vi "FollowAttacker.vi"(8 "error in (no error)":errorcluster, 9 "Game":refnum<class "Game.lvclass">, 10 "Robot":refnum<class "Robot.lvclass">, 11 "FollowAttackerSkill in":refnum<class "FollowAttackerSkill.lvclass">) -> (0 "error out":errorcluster, 2 "Robot out":refnum<class "Robot.lvclass">, 3 "FollowAttackerSkill out":refnum<class "FollowAttackerSkill.lvclass">)   [LabVIEW 2018, in "FollowAttackerSkill.lvclass"]
uses:
  FollowAttackerSkill.lvclass
  Robot_class/Robot.lvclass
  C:/Users/nicolas.oliveira/roboime/SSL_AI/Object_class/Object.lvclass
  Game_class/Game.lvclass
  Utilities_class/Utilities.lvclass
  Game_class/Game.lvclass/Game.ctl
  Team_class/Team.lvclass/Team.ctl
  Parameters_class/Parameters.lvclass/Parameters.ctl
  Events_class/Events.lvclass/Events.ctl
  Object_class/Object.lvclass/Object.ctl
  Robot_class/Robot.lvclass/Robot.ctl
  Robot_class/roles.ctl
  Object_class/Read x.vi
  Object_class/Read y.vi
  Robot_class/Read role.vi
  Robot_class/Read orientation.vi
  Game_class/Read EventsRef.vi
  Game_class/Read BallRef.vi
  Game_class/Read FieldRef.vi
  Game_class/Read OffensiveTeam.vi
  Game_class/Read Parameters.lvclass.vi
  Parameters_class/Read AttakingOurselves.vi
  Parameters_class/Read DistanceInFrontOfAttacker.vi
  Parameters_class/Read DistanceBehindAttacker.vi
  Team_class/Read RobotRef.vi
  Events_class/Read ball_inside_enemy_goalie_area.vi
  Events_class/Read ball_inside_our_goalie_area.vi
  Robot_class/Write dest_x.vi
  Robot_class/Write dest_y.vi
  Robot_class/Write dest_orientation.vi
  Robot_class/Write dest_vel.vi
  Ally_class/Ally.lvclass
  C:/Users/nicolas.oliveira/roboime/SSL_AI/Team_class/Team.lvclass
  Ball_class/Ball.lvclass
  Events_class/Events.lvclass
  Field_class/Field.lvclass
  Parameters_class/Parameters.lvclass
panel:
  out "sentido":dbl
  out "Yattacker":dbl
  out "Xattacker":dbl
  in  "Upper limit":dbl=300.0 format="%#_13g"
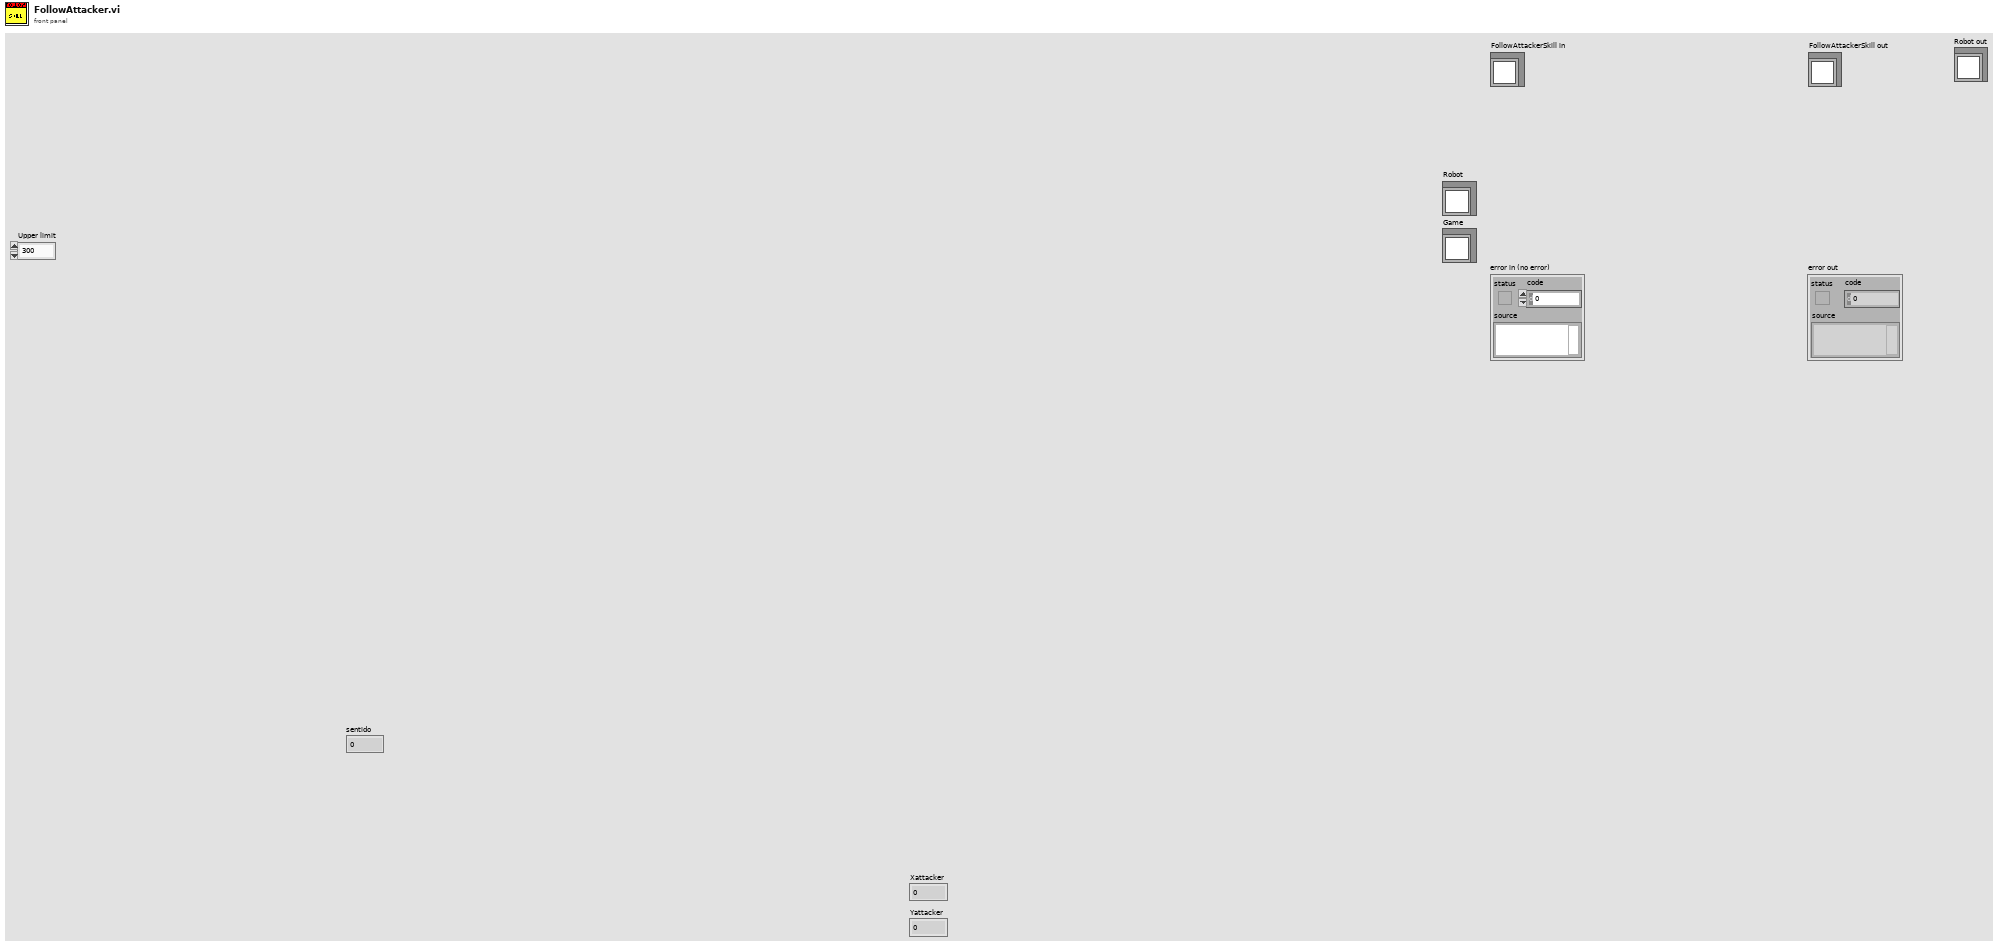
[diagram p1: front panel]
types:
  T1 = typedef "roles.ctl" = enum16{"BallOutOfField", "DefenderArea", "Duelist", "AttackerStop", "FollowAttacker", "KeeperRole", "KickPenalty", "AttackerAimGoal", "AttackerBlock", "Marker", "Halt", "Shoot", "TestRole"}
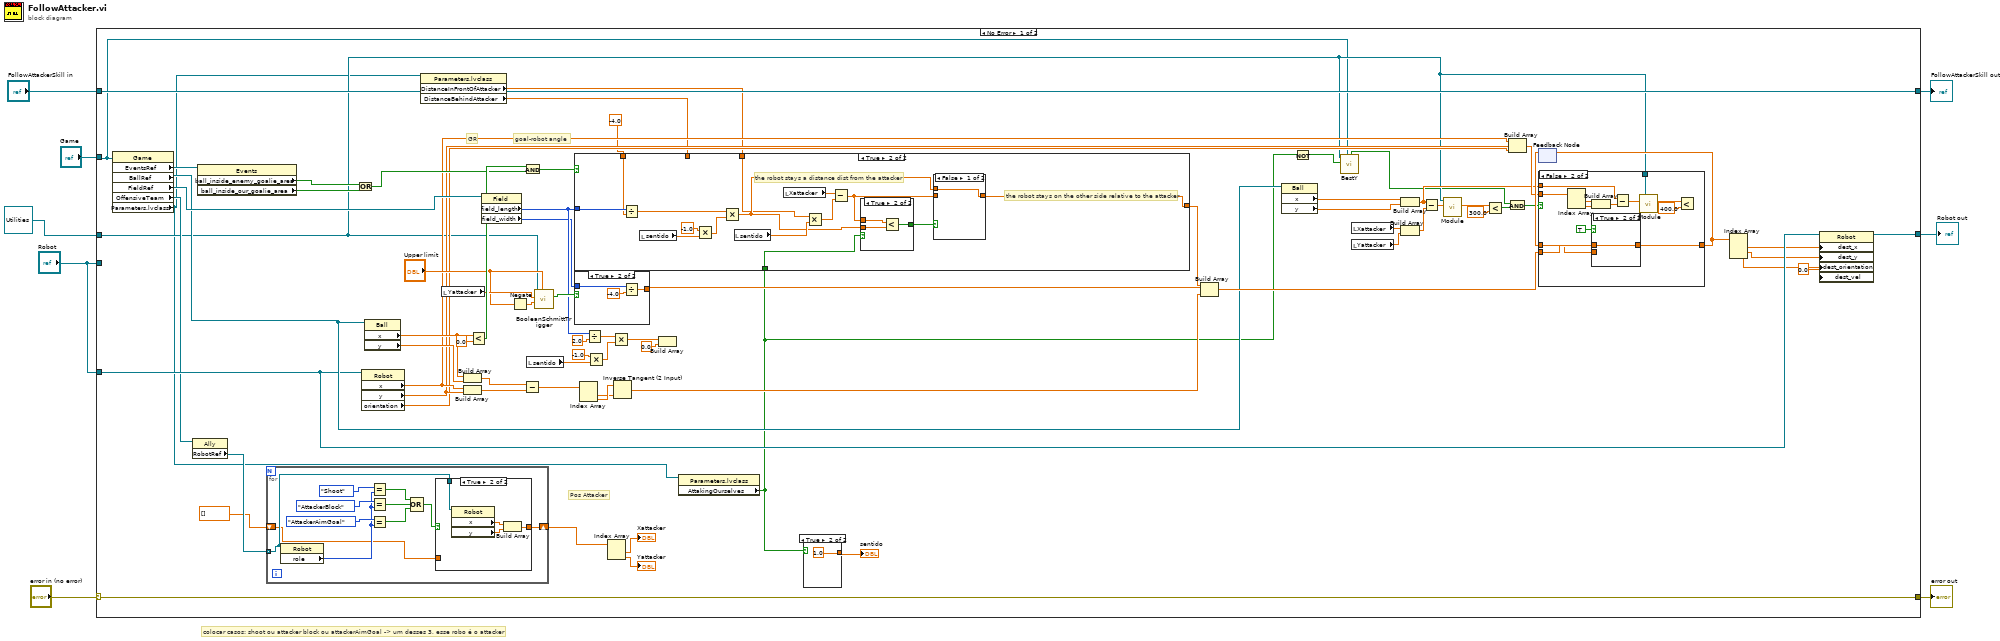
[diagram p0: block diagram]
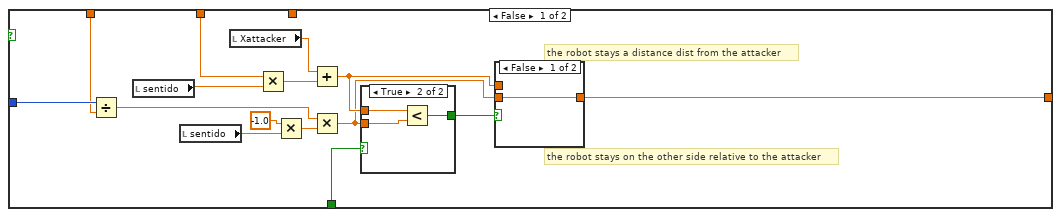
[diagram p3: hidden frame]
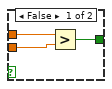
[diagram p4: hidden frame]
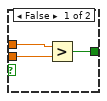
[diagram p6: hidden frame]
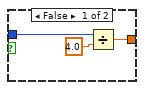
[diagram p8: hidden frame]
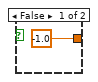
[diagram p9: hidden frame]
diagram:
  # "colocar casos: shoot ou attacker block ou attackerAimGoal -> um desses 3, esse robo é o attacker"
  n1 = case shown="No Error" "error in (no error)" {
    selector: "error in (no error)" -> [w81 w171]
    tunnel: [w81 w171] -> w7
    tunnel: [w82 w170] -> w5
    tunnel: "FollowAttackerSkill in" -> [w82 w170]
    tunnel: "Game" -> [w17 _]
    tunnel: "Robot" -> [_ w169]
    tunnel: "Robot" -> [w28 _]
    tunnel: [w30 w169] -> w1
    tunnel: refnum<class "Utilities.lvclass"> refnum ("Utilities in") -> [w18 _]
    frame No Error {
      # "Pos Attacker"
      # "GR"
      # "goal-robot angle"
      n2 = property class="Game"(reference=w17) -> ("EventsRef"=w77:refnum<class "Events.lvclass">, "BallRef"=w29:refnum<class "Ball.lvclass">, "FieldRef"=w74:refnum<class "Field.lvclass">, "OffensiveTeam"=w21:refnum<class "Ally.lvclass">, "Parameters.lvclass"=w10:refnum<class "Parameters.lvclass">)  [unwired: 1 in, 2 out]
      n3 = property class="Ally"(reference=w21) -> ("RobotRef"=w20:refnum<class "Robot.lvclass">[])  [unwired: 1 in, 2 out]
      n4 = property class="Events"(reference=w77) -> ("ball_inside_enemy_goalie_area"=w75:bool, "ball_inside_our_goalie_area"=w76:bool)  [unwired: 1 in, 2 out]
      n5 = for {
        tunnel: w20 -> [w85] mode=indexing
        shift-right: [w84] -> w15
        shift-left: dbl[] [] -> [w83]
        n6 = property class="Robot"(reference=w85) -> ("role"=w90:T1)  [unwired: 1 in, 2 out]
        n7 = Equal?(x=roles."Shoot", y=w90) -> (x = y?=w89:bool)
        n8 = Equal?(x=roles."AttackerBlock", y=w90) -> (x = y?=w88:bool)
        n9 = Equal?(x=roles."AttackerAimGoal", y=w90) -> (x = y?=w87:bool)
        n10 = Compound Arithmetic op=OR(w89, w88, w87) -> (w86:bool)
        n11 = case shown="True" w86 {
          tunnel: w85 -> [_ w98]
          tunnel: [w94 w95] -> w84
          tunnel: w83 -> [w94 _]
          frame False {
          }
          frame True {
            n12 = property class="Robot"(reference=w98) -> ("x"=w97:dbl, "y"=w96:dbl)  [unwired: 1 in, 2 out]
            n13 = Build Array(w97, w96) -> (w95:dbl[])
          }
        }
      }
      n14 = Or(x=w75, y=w76) -> (x .or. y?=w40:bool)
      n15 = property class="Robot"(reference=w28) -> ("x"=w37:dbl, "y"=w36:dbl, "orientation"=w35:dbl)  [unwired: 1 in, 2 out]
      n16 = property class="Ball"(reference=w29) -> ("x"=w39:dbl, "y"=w38:dbl)  [unwired: 1 in, 2 out]
      n17 = property class="Parameters.lvclass"(reference=w10) -> ("DistanceInFrontOfAttacker"=w12:dbl, "DistanceBehindAttacker"=w13:dbl)  [unwired: 1 in, 2 out]
      n18 = local read "Yattacker"() -> (w44:dbl)
      n19 = Build Array(w39, w38) -> (w56:dbl[])
      n20 = Build Array(w37, w36) -> (w70:dbl[])
      n21 = Less?(x=w39, y=0.0) -> (x < y?=w57:bool)
      n22 = property class="Field"(reference=w74) -> ("field_length"=w34:i32, "field_width"=w33:i32)  [unwired: 1 in, 2 out]
      n23 = Negate(x="Upper limit") -> (-x=w42:dbl)
      n24 = Subtract(x=w56, y=w70) -> (x-y=w69:dbl[])
      n25 = And(x=w57, y=w40) -> (x .and. y?=w58:bool)
      n26 = local read "sentido"() -> (w63:dbl)
      n27 = call-dynamic "BooleanSchmittTrigger.vi"("Upper limit"="Upper limit", "Lower limit"=w42, "Current Value"=w44, "Utilities in"=w18) -> ("Scmitt result"=w41:bool)  [unwired: 5 in, 2 out]
      n28 = case shown="True" w41 {
        tunnel: [w146 w149] -> w65
        tunnel: w33 -> [w145 w148]
        frame False {
          n29 = Divide(x=w145, y=4.0) -> (x/y=w146:dbl)
        }
        frame True {
          n30 = Divide(x=w148, y=-4.0) -> (x/y=w149:dbl)
        }
      }
      n31 = Index Array(array=w69) -> (element #1=w67:dbl, element #2=w68:dbl)  [unwired: 2 in]
      n32 = Divide(x=w34, y=2.0) -> (x/y=w61:dbl)
      n33 = Multiply(x=-1.0, y=w63) -> (x*y=w62:dbl)
      n34 = Index Array(array=w15) -> (element #1=→"Xattacker":dbl, element #2=→"Yattacker":dbl)  [unwired: 2 in]
      n35 = Multiply(x=w61, y=w62) -> (x*y=w60:dbl)
      n36 = Inverse Tangent (2 Input)(1:w67, 2:w68) -> (0:w73:dbl)
      n37 = Build Array(w60, 0.0 ("element")) -> ()  [unwired: 1 out]
      n38 = property class="Parameters.lvclass"(reference=w10) -> ("AttakingOurselves"=w9:bool)  [unwired: 1 in, 2 out]
      n39 = case shown="True" w58 {
        tunnel: w34 -> [w113 w136]
        tunnel: [w112 w135] -> w66
        tunnel: w13 -> [w101 _]
        tunnel: -4.0 -> [w100 w124]
        tunnel: w12 -> [_ w123]
        tunnel: w9 -> [w99 w122]
        frame False {
          # "the robot stays on the other side relative to the attacker"
          # "the robot stays a distance dist from the attacker"
          n40 = Divide(x=w113, y=w100) -> (x/y=w111:dbl)
          n41 = local read "sentido"() -> (w105:dbl)
          n42 = local read "sentido"() -> (w108:dbl)
          n43 = local read "Xattacker"() -> (w110:dbl)
          n44 = Multiply(x=w101, y=w105) -> (x*y=w109:dbl)
          n45 = Multiply(x=-1.0, y=w108) -> (x*y=w107:dbl)
          n46 = Add(x=w110, y=w109) -> (x+y=w104:dbl)
          n47 = Multiply(x=w111, y=w107) -> (x*y=w103:dbl)
          n48 = case shown="True" w99 {
            tunnel: w104 -> [w116 w118]
            tunnel: w103 -> [w115 w119]
            tunnel: [w114 w117] -> w102
            frame False {
              n49 = Greater?(x=w116, y=w115) -> (0:w114:bool)
            }
            frame True {
              n50 = Less?(x=w118, y=w119) -> (x < y?=w117:bool)
            }
          }
          n51 = case shown="False" w102 {
            tunnel: [w120 w121] -> w112
            tunnel: w104 -> [_ w121]
            tunnel: w103 -> [w120 _]
            frame False {
            }
            frame True {
            }
          }
        }
        frame True {
          # "the robot stays on the other side relative to the attacker"
          # "the robot stays a distance dist from the attacker"
          n52 = Divide(x=w136, y=w124) -> (x/y=w134:dbl)
          n53 = local read "sentido"() -> (w131:dbl)
          n54 = Multiply(x=-1.0, y=w131) -> (x*y=w130:dbl)
          n55 = Multiply(x=w134, y=w130) -> (x*y=w126:dbl)
          n56 = local read "sentido"() -> (w128:dbl)
          n57 = local read "Xattacker"() -> (w133:dbl)
          n58 = Multiply(x=w123, y=w128) -> (x*y=w132:dbl)
          n59 = Subtract(x=w133, y=w132) -> (x-y=w127:dbl)
          n60 = case shown="True" w122 {
            tunnel: w127 -> [w139 w141]
            tunnel: w126 -> [w138 w142]
            tunnel: [w137 w140] -> w125
            frame False {
              n61 = Greater?(x=w139, y=w138) -> (0:w137:bool)
            }
            frame True {
              n62 = Less?(x=w141, y=w142) -> (x < y?=w140:bool)
            }
          }
          n63 = case shown="False" w125 {
            tunnel: [w143 w144] -> w135
            tunnel: w127 -> [_ w144]
            tunnel: w126 -> [w143 _]
            frame False {
            }
            frame True {
            }
          }
        }
      }
      n64 = case shown="True" w9 {
        tunnel: [-1.0 1.0] -> w80
        frame False {
        }
        frame True {
        }
      }
      "sentido" <- w80
      n65 = Build Array(w66, w65, w73) -> (w55:dbl[])
      n66 = property class="Ball"(reference=w29) -> ("x"=w32:dbl, "y"=w31:dbl)  [unwired: 1 in, 2 out]
      n67 = Not(x=w9) -> (.not. x?=w19:bool)
      n68 = call-dynamic "BestY.vi"("Game"=w17, "inimigos"=w19, "Utilities in"=w18) -> ("Eclipse"=w16:bool)  [unwired: 3 in, 5 out]
      n69 = local read "Xattacker"() -> (w52:dbl)
      n70 = local read "Yattacker"() -> (w51:dbl)
      n71 = Build Array(w32, w31) -> (w45:dbl[])
      n72 = Build Array(w52, w51) -> (w50:dbl[])
      n73 = Subtract(x=w45, y=w50) -> (x-y=w23:dbl[])
      n74 = call-dynamic "Module.vi"("2D vector"=w23, "Utilities in"=w18) -> ("Modulo"=w22:dbl)  [unwired: 7 in, 2 out]
      n75 = Less?(x=w22, y=300.0 ("x")) -> (x < y?=w48:bool)
      n76 = And(x=w16, y=w48) -> (x .and. y?=w49:bool)
      n77 = Build Array(w37, w36, w35) -> (w46:dbl[])
      n78 = feedback #1() -> (w53:dbl[])  [unwired: 1 in]
      n79 = case shown="False" w49 {
        tunnel: w55 -> [_ w159]
        tunnel: [w153 w160] -> w54
        tunnel: w53 -> [w153 w158]
        tunnel: w46 -> [_ w166]
        tunnel: w45 -> [_ w163]
        tunnel: w18 -> [_ w154]
        frame True {
        }
        frame False {
          n80 = Index Array(array=w166) -> (element #1=w165:dbl, element #2=w164:dbl)  [unwired: 2 in]
          n81 = Build Array(w165, w164) -> (w162:dbl[])
          n82 = case shown="True" TRUE {
            tunnel: [w167 w168] -> w160
            tunnel: w159 -> [_ w168]
            tunnel: w158 -> [w167 _]
            frame False {
            }
            frame True {
            }
          }
          n83 = Subtract(x=w163, y=w162) -> (x-y=w156:dbl[])
          n84 = call-dynamic "Module.vi"("2D vector"=w156, "Utilities in"=w154) -> ("Modulo"=w155:dbl)  [unwired: 7 in, 2 out]
          n85 = Less?(x=w155, y=400.0) -> ()  [unwired: 1 out]
        }
      }
      n86 = feedback-in #1(w54) -> ()
      n87 = Index Array(array=w54) -> (element #1=w27:dbl, element #2=w26:dbl, element #3=w25:dbl)  [unwired: 3 in]
      n88 = property class="Robot"(reference=w28, "dest_x"=w27, "dest_y"=w26, "dest_orientation"=w25, "dest_vel"=0.0) -> (reference out=w30:refnum<class "Robot.lvclass">)  [unwired: 1 in, 1 out]
    }
    frame Error {
    }
  }
  "error out" <- w7
  "FollowAttackerSkill out" <- w5
  "Robot out" <- w1
